vi "Facade 1.vi"(0 "Data In":T4, 2 "Display State In":T2, 3 "Container State":T3) -> (6 "Data Out":T4, 7 "Display State Out":T2, 8 "Action":T1)   [LabVIEW 2012, in "Intellisense Xcontrol.xctl"]
uses:
  Intellisense Xcontrol.xctl
  Data 1.ctl
  <vilib>/_xctls/Container State.ctl
  State 1.ctl
  <vilib>/_xctls/Action.ctl
  <vilib>/event_ctls.llb/eventvkey.ctl
  <vilib>/_xctls/XControlSupport.lvlib
panel:
  in  "String":string
  # "1. Drop the controls that make up the appearance\nof the XControl here.\n\n2. Resize the window to fit the controls\n\n3. If the XControl is of fixed size,  make the \n window not resizable from VI Properties->Window Appearance.\n\n4. If you want the controls to automatically size when the XControl sizes, check  \"Scale all objects on front panel when window resizes\" in File->VI Properties->Window Size page.\n\n5. Show the block diagram and handle events for the controls on this panel."
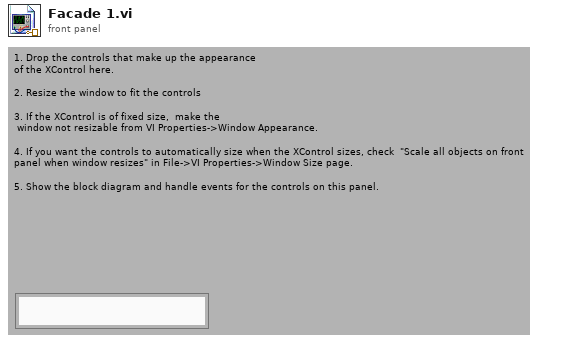
[diagram p1: front panel]
types:
  T1 = typedef "XControlSupport.lvlib/Action.ctl" = cluster{"Data Changed?":bool, "State Changed?":bool, "Action Name":string}
  T2 = typedef "Intellisense Xcontrol.xctl/State 1.ctl" = cluster{"Keyword Array":string[], "Auto-Complete On/Off":bool, "Delimiter":string}
  T3 = typedef "XControlSupport.lvlib/Container State.ctl" = cluster{"Indicator?":bool, "Run Mode?":bool, " Refnum":refnum<vi>}
  T4 = typedef "Intellisense Xcontrol.xctl/Data 1.ctl" = string
  T5 = typedef "eventvkey.ctl" = enum16{"ASCII", "Enter", "Return", "Shift", "Ctrl", "Alt", "Cmd", "Opt", "Caps", "NumLock", "Clear", "Break", "Up", "Down", "Left", "Right", "Insert", "Delete", "Home", "End", "PageUp", "PageDown", "Escape", "Help", "Pause", "ScrollLock", "F1", "F2", "F3", "F4", "F5", "F6", "F7", "F8", "F9", "F10", "F11", "F12", "F13", "F14", "F15", "F16", "F17", "F18", "F19", "F20", "F21", "F22", "F23", "F24", "Play", "VolumeUp", "VolumeDown", "Mute", "Two Byte Char"}
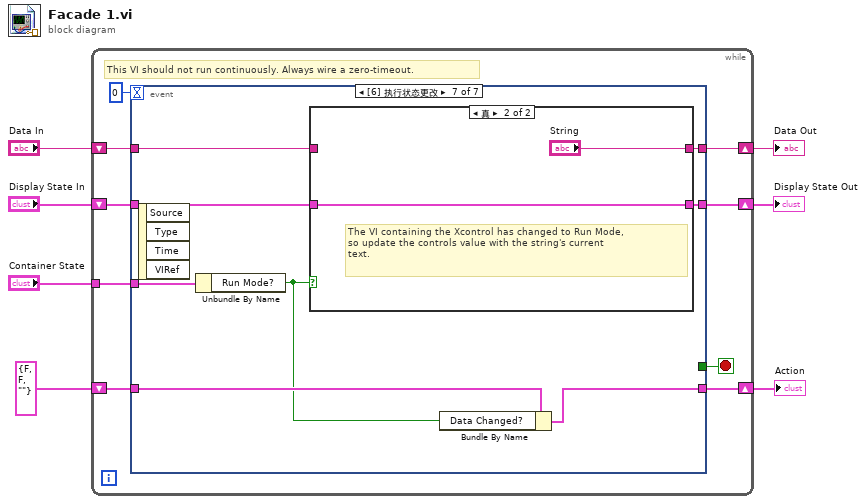
[diagram p0: block diagram]
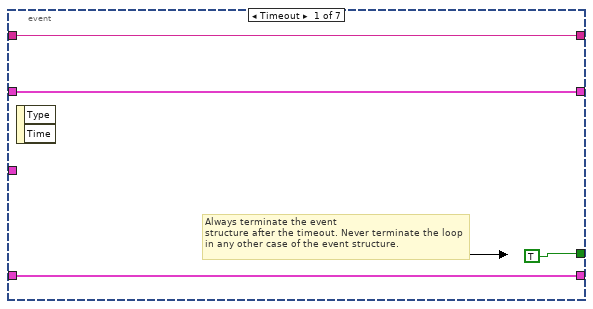
[diagram p2: hidden frame]
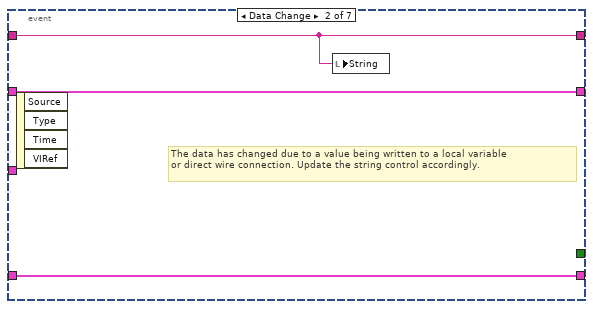
[diagram p3: hidden frame]
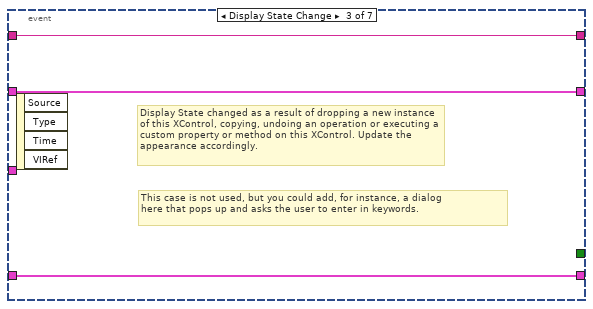
[diagram p4: hidden frame]
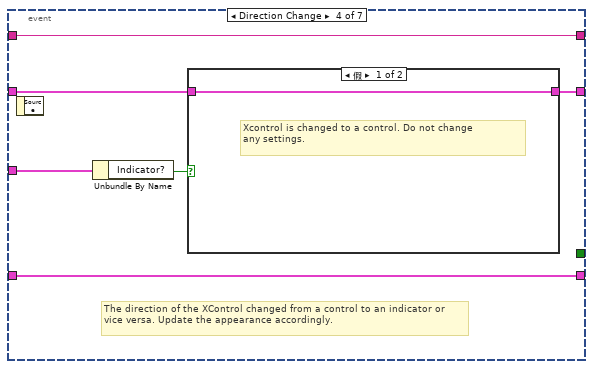
[diagram p5: hidden frame]
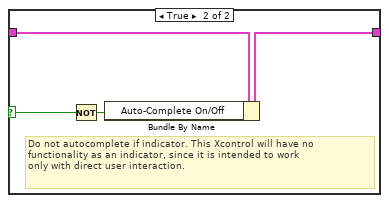
[diagram p6: hidden frame]
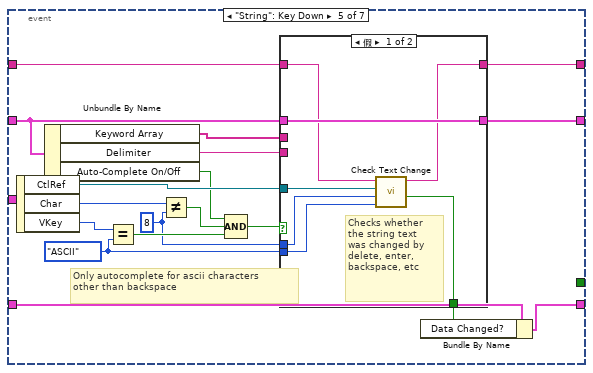
[diagram p7: hidden frame]
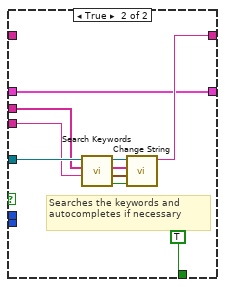
[diagram p8: hidden frame]
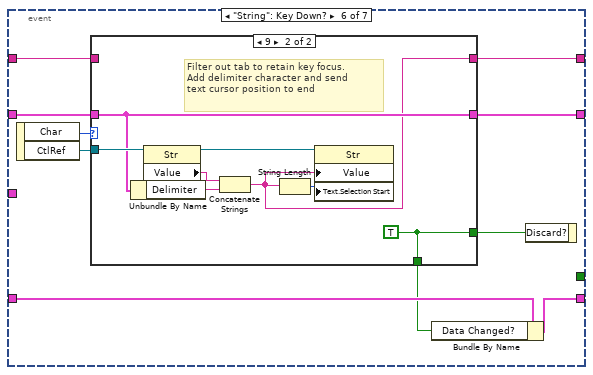
[diagram p9: hidden frame]
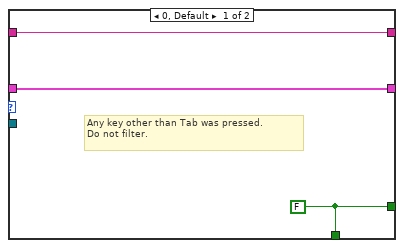
[diagram p10: hidden frame]
diagram:
  n1 = while {
    shift-right: [w15] -> w4
    shift-left: "Display State In" -> [w16]
    tunnel: "Container State" -> [w12]
    shift-right: [w10] -> w7
    shift-left: "Data In" -> [w11]
    shift-right: [w8] -> w2
    shift-left: T1 {"Data Changed?"=FALSE, "State Changed?"=FALSE, "Action Name"=""} ("Action") -> [w9]
    stop <- w14 stop-if-true
    # "This VI should not run continuously. Always wire a zero-timeout."
    n2 = event shown="[6] 执行状态更改" {
      selector: _ -> [_ _ _ _ _ _ _]
      dyn-events: _ -> [_ _ _ _ _ _ _]
      timeout: 0 -> [_ _ _ _ _ _ _]
      tunnel: w16 -> [w18 w23 w26 w29 w49 w74 w96]
      tunnel: [w18 w23 w26 w28 w48 w73 w95] -> w15
      tunnel: [TRUE _ _ _ _ _ _] -> w14
      tunnel: w12 -> [_ _ _ w32 _ _ w101]
      tunnel: w11 -> [w17 w21 w25 w31 w47 w76 w97]
      tunnel: [w17 w21 w25 w31 w51 w75 w100] -> w10
      tunnel: [w19 w22 w24 w30 w54 w78 w98] -> w8
      tunnel: w9 -> [w19 w22 w24 w30 w55 w79 w99]
      event Timeout {
        # "Always terminate the event\nstructure after the timeout. Never terminate the loop in any other case of the event structure."
        n3 = event-data() -> ()  [unwired: 1 in, 2 out]
      }
      event Data Change {
        # "The data has changed due to a value being written to a local variable\nor direct wire connection. Update the string control accordingly."
        n4 = event-data() -> ()  [unwired: 1 in, 4 out]
        n5 = local write "String"(w21) -> ()
      }
      event Display State Change {
        # "This case is not used, but you could add, for instance, a dialog\nhere that pops up and asks the user to enter in keywords."
        # "Display State changed as a result of dropping a new instance of this XControl, copying, undoing an operation or executing a custom property or method on this XControl. Update the appearance accordingly."
        n6 = event-data() -> ()  [unwired: 1 in, 4 out]
      }
      event Direction Change {
        # "The direction of the XControl changed from a control to an indicator or vice versa. Update the appearance accordingly."
        n7 = event-data() -> ()  [unwired: 1 in, 1 out]
        n8 = Unbundle By Name(w32) -> ("Indicator?"=w27:bool)
        n9 = case shown="假" w27 {
          selector: w27 -> [_ w34]
          tunnel: w29 -> [w33 w37]
          tunnel: [w33 w35] -> w28
          frame False {
            # "Xcontrol is changed to a control. Do not change\nany settings."
          }
          frame True {
            # "Do not autocomplete if indicator. This Xcontrol will have no\nfunctionality as an indicator, since it is intended to work\nonly with direct user interaction."
            n10 = Not(x=w34) -> (.not. x?=w36:bool)
            n11 = Bundle By Name(cluster=w37, "Auto-Complete On/Off"=w36) -> (w35:T2)
          }
        }
      }
      event "String": Key Down {
        w38 = i16 8 ("Char")
        w39 = eventvkey."ASCII" ("VKey")
        # "Only autocomplete for ascii characters\nother than backspace"
        n12 = event-data() -> ("CtlRef"=w53:refnum<vi>, "Char"=w42:i16, "VKey"=w43:T5)  [unwired: 1 in]
        n13 = Unbundle By Name(w49) -> ("Keyword Array"=w52:string[], "Delimiter"=w46:string, "Auto-Complete On/Off"=w45:bool)
        n14 = Equal?(x=w43, y=w39) -> (x = y?=w40:bool)
        n15 = Not Equal?(x=w42, y=w38) -> (x != y?=w41:bool)
        n16 = Compound Arithmetic op=AND(w45, w41, w40) -> (w44:bool)
        n17 = case shown="假" w44 {
          tunnel: w53 -> [w60 w72]
          tunnel: w52 -> [_ w66]
          tunnel: [w59 w70] -> w51
          tunnel: w46 -> [_ w69]
          tunnel: [w56 TRUE ("Data Changed?")] -> w50
          tunnel: w49 -> [w62 w63]
          tunnel: [w62 w63] -> w48
          tunnel: w47 -> [w61 _]
          tunnel: w39 -> [w57 _]
          tunnel: w38 -> [w58 _]
          frame False {
            # "Checks whether\nthe string text\nwas changed by\ndelete, enter,\nbackspace, etc"
            n18 = call "Check Text Change.vi"("VKey"=w57, "Char"=w58, "Str Refnum"=w60, "Data In"=w61) -> ("Text Changed?"=w56:bool, "Data Out"=w59:string)  [unwired: 6 in]
          }
          frame True {
            # "Searches the keywords and\nautocompletes if necessary"
            n19 = call "Search Keywords.vi"("Delimiter"=w69, "Keyword Array"=w66, "Str Refnum"=w72) -> ("Match Found?"=w65:bool, "Match Cluster"=w68:cluster{"Item Index":i32, "Offset":i32}, "Keyword Array Out"=w67:string[], "Str Refnum Out"=w71:refnum<vi>)  [unwired: 5 in]
            n20 = call "Change String.vi"("AutoComplete?"=w65, "Match Cluster"=w68, "Keyword Array"=w67, "String Refnum"=w71) -> ("String Value"=w70:string)  [unwired: 7 in]
          }
        }
        n21 = Bundle By Name(cluster=w55, "Data Changed?"=w50) -> (w54:T1)
      }
      event "String": Key Down? {
        n22 = event-data() -> ("Char"=w82:i16, "CtlRef"=w81:refnum<vi>)  [unwired: 1 in]
        n23 = case shown="9" w82 {
          tunnel: w81 -> [_ w92]
          tunnel: [w85 w93] -> w80
          tunnel: [w85 w93] -> w77
          tunnel: w76 -> [w84 _]
          tunnel: [w84 w86] -> w75
          tunnel: w74 -> [w83 w88]
          tunnel: [w83 w88] -> w73
          frame 0, Default {
            w85 = FALSE
            # "Any key other than Tab was pressed.\nDo not filter."
          }
          frame 9 {
            w93 = TRUE
            # "Filter out tab to retain key focus.\nAdd delimiter character and send\ntext cursor position to end"
            n24 = Unbundle By Name(w88) -> ("Delimiter"=w87:string)
            n25 = property class="Str"(reference=w92) -> (reference out=w91:refnum<vi>, "Value"=w90:string)  [unwired: 1 in, 1 out]
            n26 = Concatenate Strings(w90, w87) -> (w86:string)
            n27 = String Length(string=w86) -> (length=w89:i32)
            n28 = property class="Str"(reference=w91, "Value"=w86, "Text.Selection Start"=w89) -> ()  [unwired: 1 in, 2 out]
          }
        }
        n29 = Bundle By Name(cluster=w79, "Data Changed?"=w77) -> (w78:T1)
        n30 = event-data("Discard?"=w80) -> ()  [unwired: 1 in, 1 out]
      }
      event Exec State Change {
        n31 = event-data() -> ()  [unwired: 1 in, 4 out]
        n32 = Unbundle By Name(w101) -> ("Run Mode?"=w94:bool)
        n33 = case shown="真" w94 {
          tunnel: [w103 "String"] -> w100
          tunnel: w97 -> [w103 _]
          tunnel: w96 -> [w102 w104]
          tunnel: [w102 w104] -> w95
          frame False {
          }
          frame True {
            # "The VI containing the Xcontrol has changed to Run Mode,\nso update the controls value with the string's current\ntext."
          }
        }
        n34 = Bundle By Name(cluster=w99, "Data Changed?"=w94) -> (w98:T1)
      }
    }
  }
  "Display State Out" <- w4
  "Data Out" <- w7
  "Action" <- w2
